vi "Set DDG Gate Time.vi"(10 "uiWidth":cluster{}, 11 "uiDelay":cluster{}) -> (3 "function return":u32)   [LabVIEW 2018, in "Copy of Andor SDK.lvlib"]
doc: "EXPNETTYPE unsigned int WINAPI SetDDGGateTime(at_u64 uiDelay, at_u64 uiWidth);"
uses:
  Copy of Andor SDK.lvlib
  <userlib>/Andor SDK/ATMCD32D.dll
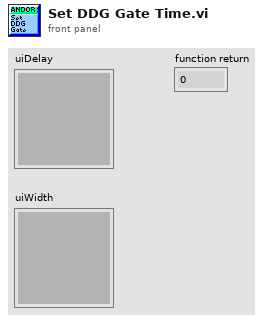
[diagram p1: front panel]
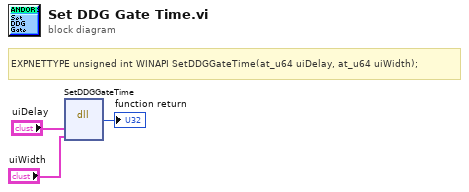
[diagram p0: block diagram]
diagram:
  # "EXPNETTYPE unsigned int WINAPI SetDDGGateTime(at_u64 uiDelay, at_u64 uiWidth);"
  n1 = dll-call lib="C:/Program Files (x86)/National Instruments/LabVIEW 2018/user.lib/Andor SDK/ATMCD32D.*" fn="SetDDGGateTime"("uiDelay"="uiDelay", "uiWidth"="uiWidth") -> (→"function return":u32)  [unwired: 5 in, 2 out]
